vi "load config data.vi"(8 "error in (no error)":errorcluster, 11 "Sim Camera Driver in":refnum<class "Sim Camera Driver.lvclass">) -> (0 "error out":errorcluster, 3 "Sim Camera Driver out":refnum<class "Sim Camera Driver.lvclass">)   [LabVIEW 2022 SP3, in "Sim Camera Driver.lvclass"]
uses:
  Sim Camera Driver.lvclass
  Sim Camera Driver.lvclass/Sim Camera Driver.ctl
  cfbc573d-5e92-4fd1-b197-78dee3d8c778.vi
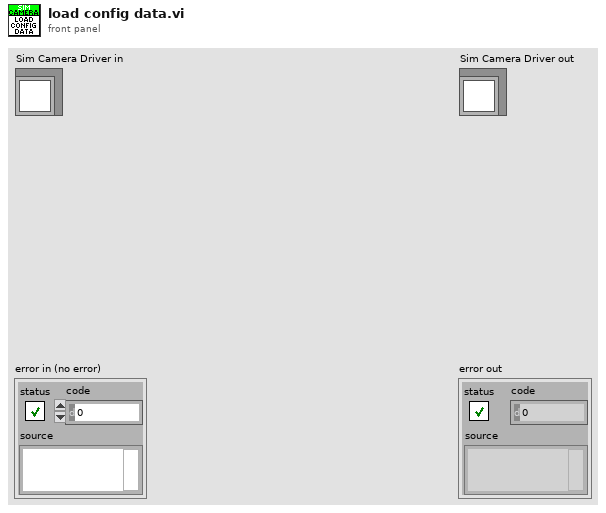
[diagram p1: front panel]
types:
  T1 = typedef "Sim Camera Driver.lvclass/Settings.ctl" = cluster{"Sim Image":path}
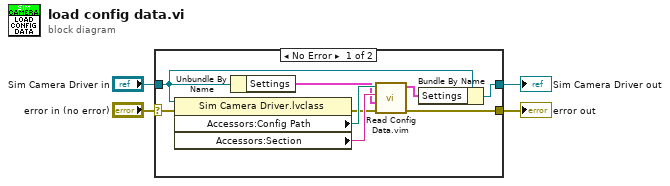
[diagram p0: block diagram]
diagram:
  n1 = case shown="No Error" "error in (no error)" {
    selector: "error in (no error)" -> [w6 w15]
    tunnel: [w5 w15] -> w4
    tunnel: [w8 w14] -> w3
    tunnel: "Sim Camera Driver in" -> [w7 w14]
    frame No Error {
      n2 = property class="Sim Camera Driver.lvclass"(reference=w7, error in=w6) -> (error out=w9:errorcluster, "Accessors:Config Path"=w13:path, "Accessors:Section"=w12:string)  [unwired: 1 out]
      n3 = Unbundle By Name(w7) -> ("Settings"=w11:T1)
      n4 = call "Read Config Data.vim"("error in (no error)"=w9, "Section Formatted Cluster Type"=w11, "Section"=w12, "Config Path"=w13) -> ("error out"=w5:errorcluster, "Section Formatted Cluster Type 2"=w10:T1)  [unwired: 6 in]
      n5 = Bundle By Name(cluster=w7, "Settings"=w10) -> (w8:refnum<class "Sim Camera Driver.lvclass">)
    }
    frame Error {
    }
  }
  "error out" <- w4
  "Sim Camera Driver out" <- w3
